vi "Apply CAN Configuration.vi"(7 "Restart (T)":bool=TRUE, 8 "error in (no error)":errorcluster, 10 "CAN Settings":T1={"Box ID"=1, "Publish Period (ms)"=5}, 11 "Ethernet in":refnum<class "ENET_BS120x.lvclass">) -> (0 "error out":errorcluster, 3 "Ethernet out":refnum<class "ENET_BS120x.lvclass">)   [LabVIEW 2021, in "BS120x Driver.lvlib" / "ENET_BS120x.lvclass"]
doc: "Sends the configuration updates to the Battery Simulator 1200. Changes will not be applied until after the unit is restarted. To apply multilple configuration settings in one set, set <b>Restart</b> to false on all Settings VIs except the last one.\n(c) 2019 Bloomy Controls, Inc. All rights reserved."
uses:
  ENET_BS120x.lvclass
  TypeDefs/CAN Settings.ctl
  ENET_BS120x.lvclass/ENET_BS120x.ctl
  BS120x.lvclass
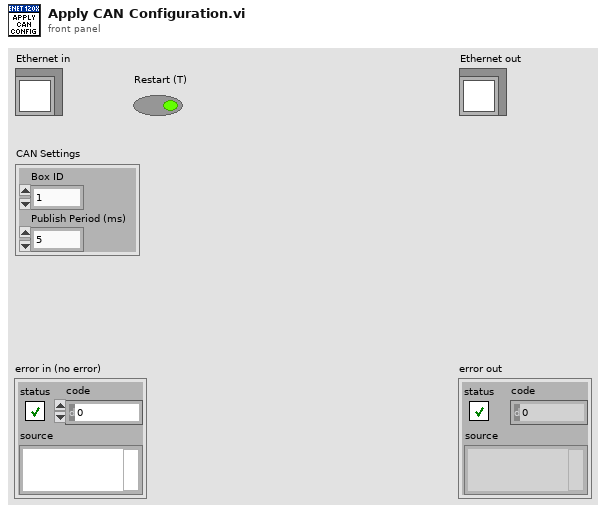
[diagram p1: front panel]
types:
  T1 = typedef "BS120x Driver.lvlib/BS120x.lvclass/CAN Settings.ctl" = cluster{"Box ID":i32, "Publish Period (ms)":i32}
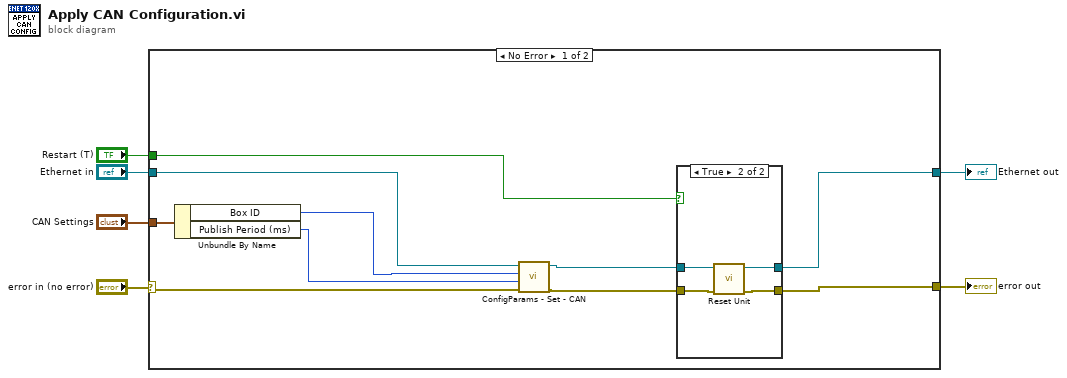
[diagram p0: block diagram]
diagram:
  n1 = case shown="No Error" "error in (no error)" {
    selector: "error in (no error)" -> [w11 w24]
    tunnel: [w15 w24] -> w5
    tunnel: [w16 w23] -> w3
    tunnel: "Ethernet in" -> [w10 w23]
    tunnel: "CAN Settings" -> [w14 _]
    tunnel: "Restart (T)" -> [w13 _]
    frame No Error {
      n2 = Unbundle By Name(w14) -> ("Box ID"=w8:i32, "Publish Period (ms)"=w7:i32)
      n3 = call-dynamic "ConfigParams - Set - CAN.vi"("error in (no error)"=w11, "WritePeriod_ms"=w7, "BoxID"=w8, "Ethernet in"=w10) -> ("error out"=w12:errorcluster, "Ethernet out"=w9:refnum<class "ENET_BS120x.lvclass">)  [unwired: 6 in]
      n4 = case shown="True" w13 {
        tunnel: [w18 w22] -> w15
        tunnel: [w17 w21] -> w16
        tunnel: w12 -> [w18 w20]
        tunnel: w9 -> [w17 w19]
        frame False {
        }
        frame True {
          n5 = call-dynamic "Reset Unit.vi"("error in (no error)"=w20, "Ethernet in"=w19) -> ("error out"=w22:errorcluster, "Ethernet out"=w21:refnum<class "ENET_BS120x.lvclass">)  [unwired: 8 in]
        }
      }
    }
    frame Error {
    }
  }
  "error out" <- w5
  "Ethernet out" <- w3
